vi "Configure Trigger (Delay).vi"(0 "VISA resource name":refnum<visa-resource-name>, 1 "Delay Time (3E-8 s)":dbl=3e-08, 2 "Event Number (0)":i32, 5 "Trigger Source (1: Channel1)":i32(ring)=1 items=["Channel1"=1, "Channel2"=2, "Channel3"=3, "Channel4"=4, "DIG0"=20, "DIG1"=21, "DIG2"=22, "DIG3"=23, "DIG4"=24, "DIG5"=25, "DIG6"=26, "DIG7"=27, "DIG8"=28, "DIG9"=29, "DIG10"=30, "DIG11"=31, "DIG12"=32, "DIG13"=33, "DIG14"=34, "DIG15"=35], 7 "Arming Slope (0: Negative)":i32(ring) items=["Negative", "Positive"], 9 "Delay Trigger Mode (0: Trigger After Time)":i32(ring) items=["Trigger After Time", "Trigger on nth Event"], 11 "error in (no error)":errorcluster, 12 "Delay Trigger Slope (0: Negative)":i32(ring) items=["Negative", "Positive"], 13 "Event Slope (0: Negative)":i32(ring) items=["Negative", "Positive"]) -> (4 "VISA resource name out":refnum<visa-resource-name>, 15 "error out":errorcluster)   [LabVIEW 2020, in "Agilent 90000 Series.lvlib"]
doc: "Configures the delay trigger parameters."
uses:
  Agilent 90000 Series.lvlib
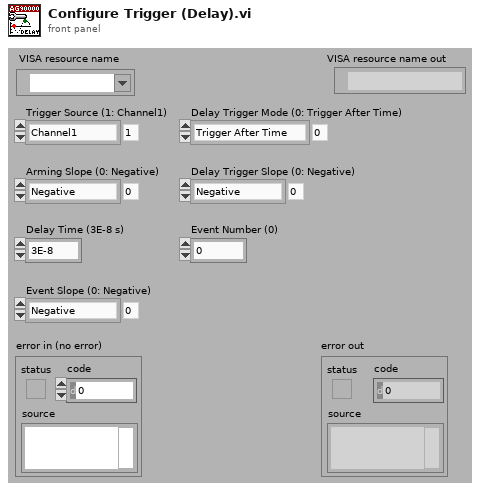
[diagram p1: front panel]
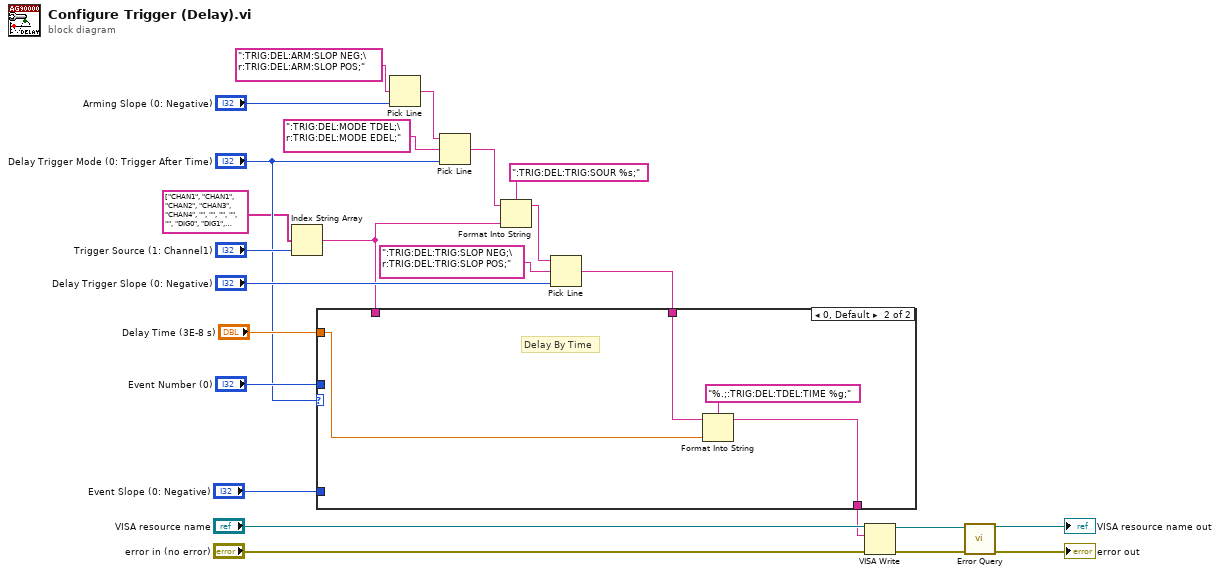
[diagram p0: block diagram]
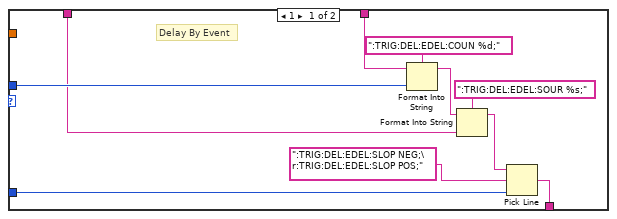
[diagram p2: hidden frame]
diagram:
  n1 = Index String Array(1:"Trigger Source (1: Channel1)", 2:string[] ["CHAN1", "CHAN1", "CHAN2", "CHAN3", "CHAN4", "", "", "", "", "", "DIG0", "DIG1", "DIG2", "DIG3", "DIG4", "DIG5", "DIG6", "DIG7", "DIG8", "DIG9", "DIG0", "DIG1", "DIG2", "DIG3", "DIG4", "DIG5", "DIG6", "DIG7", "DIG8", "DIG9", "DIG10", "DIG11", "DIG12", "DIG13", "DIG14", "DIG15"]) -> (0:w7:string)  [unwired: 1 out]
  n2 = Pick Line(multi-line string=":TRIG:DEL:ARM:SLOP NEG;\r:TRIG:DEL:ARM:SLOP POS;", line index="Arming Slope (0: Negative)") -> (output string=w22:string)  [unwired: 1 out]
  n3 = Pick Line(string ("")=w22, multi-line string=":TRIG:DEL:MODE TDEL;\r:TRIG:DEL:MODE EDEL;", line index="Delay Trigger Mode (0: Trigger After Time)") -> (output string=w4:string)
  n4 = Format Into String(format string=":TRIG:DEL:TRIG:SOUR %s;", initial string=w4, w7) -> (resulting string=w6:string)  [unwired: 1 in, 1 out]
  n5 = Pick Line(string ("")=w6, multi-line string=":TRIG:DEL:TRIG:SLOP NEG;\r:TRIG:DEL:TRIG:SLOP POS;", line index="Delay Trigger Slope (0: Negative)") -> (output string=w3:string)
  n6 = case shown="0, Default" "Delay Trigger Mode (0: Trigger After Time)" {
    tunnel: "Delay Time (3E-8 s)" -> [_ w37]
    tunnel: "Event Number (0)" -> [w33 _]
    tunnel: "Event Slope (0: Negative)" -> [w30 _]
    tunnel: w7 -> [w28 _]
    tunnel: [w26 w35] -> w5
    tunnel: w3 -> [w25 w36]
    frame 1 {
      # "Delay By Event"
      n7 = Format Into String(format string=":TRIG:DEL:EDEL:COUN %d;", initial string=w25, w33) -> (resulting string=w32:string)  [unwired: 1 in, 1 out]
      n8 = Format Into String(format string=":TRIG:DEL:EDEL:SOUR %s;", initial string=w32, w28) -> (resulting string=w27:string)  [unwired: 1 in, 1 out]
      n9 = Pick Line(string ("")=w27, multi-line string=":TRIG:DEL:EDEL:SLOP NEG;\r:TRIG:DEL:EDEL:SLOP POS;", line index=w30) -> (output string=w26:string)
    }
    frame 0, Default {
      # "Delay By Time"
      n10 = Format Into String(format string="%.;:TRIG:DEL:TDEL:TIME %g;", initial string=w36, w37) -> (resulting string=w35:string)  [unwired: 1 in, 1 out]
    }
  }
  n11 = VISA Write(VISA resource name="VISA resource name", write buffer=w5, error in (no error)="error in (no error)") -> (VISA resource name out=w13:refnum<visa-resource-name>, error out=w12:errorcluster)  [unwired: 1 out]
  n12 = call "Error Query.vi"("error in (no error)"=w12, "VISA resource name"=w13) -> ("error out"=→"error out":errorcluster, "VISA resource name out"=→"VISA resource name out":refnum<visa-resource-name>)  [unwired: 8 out]
